vi "Configure Generator Output.vi"(8 "error in (no error)":errorcluster, 9 "Waveform Generator Output Mode (0: Normal)":i32(ring) items=["Normal", "Single"], 10 "Waveform Generator Number (1: Waveform Generator 1)":i32(ring)=1 items=["Waveform Generator 1"=1, "Waveform Generator 2"=2], 11 "VISA resource name":refnum<visa-resource-name>) -> (0 "error out":errorcluster, 3 "VISA resource name out":refnum<visa-resource-name>)   [LabVIEW 2023, in "Keysight-DSQx3014T.lvlib"]
doc: "Specifies the output mode of the waveform generator. Use this VI to enable single-cycle output for the waveform generator."
uses:
  Keysight-DSQx3014T.lvlib
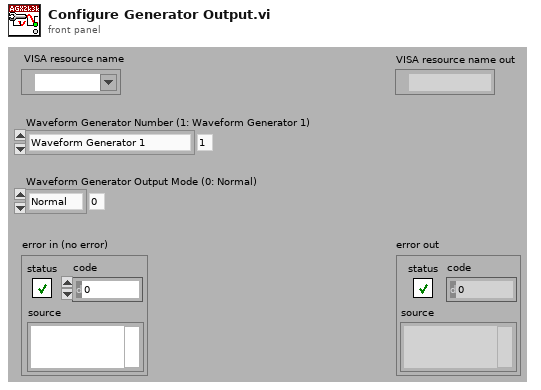
[diagram p1: front panel]
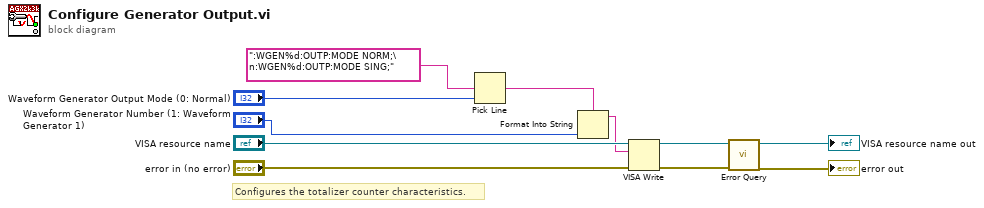
[diagram p0: block diagram]
diagram:
  # "Configures the totalizer counter characteristics."
  n1 = Pick Line(multi-line string=":WGEN%d:OUTP:MODE NORM;\n:WGEN%d:OUTP:MODE SING;", line index="Waveform Generator Output Mode (0: Normal)") -> (output string=w2:string)  [unwired: 1 in]
  n2 = Format Into String(format string=w2, "Waveform Generator Number (1: Waveform Generator 1)") -> (resulting string=w3:string)  [unwired: 2 in, 1 out]
  n3 = VISA Write(VISA resource name="VISA resource name", write buffer=w3, error in (no error)="error in (no error)") -> (VISA resource name out=w11:refnum<visa-resource-name>, error out=w10:errorcluster)  [unwired: 1 out]
  n4 = call "Error Query.vi"("error in (no error)"=w10, "VISA resource name"=w11) -> ("error out"=→"error out":errorcluster, "VISA resource name out"=→"VISA resource name out":refnum<visa-resource-name>)  [unwired: 8 out]
